vi "InitSerialPort.vi"(1 "default resource name":refnum<visa-resource-name>) -> (0 "VISA resource name out":refnum<visa-resource-name>)   [LabVIEW 2010]
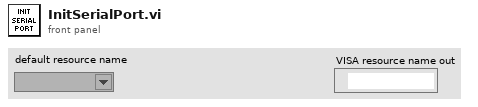
[diagram p1: front panel]
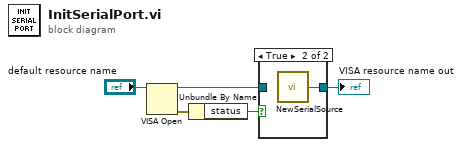
[diagram p0: block diagram]
diagram:
  n1 = VISA Open(VISA resource name="default resource name") -> (VISA resource name=w3:refnum<visa-resource-name>, error out=w2:errorcluster)  [unwired: 4 in]
  n2 = Unbundle By Name(w2) -> ("status"=w1:bool)
  n3 = case shown="True" w1 {
    tunnel: [w6 w7] -> w4
    tunnel: w3 -> [w6 _]
    frame False {
    }
    frame True {
      n4 = call "NewSerialSource.vi"() -> ("Select Source 2"=w7:refnum<visa-resource-name>)  [unwired: 1 in]
    }
  }
  "VISA resource name out" <- w4
